vi "New Items.vi"(8 "error in (no error)":errorcluster, 10 "New Items":refnum<class "BetterItem.lvclass">[](array[class]), 11 "BetterTreeHandle in":refnum<class "BetterTreeHandle.lvclass">) -> (0 "error out":errorcluster, 3 "BetterTreeHandle out":refnum<class "BetterTreeHandle.lvclass">)   [LabVIEW 2020, in "BetterDragAndDrop.lvlib" / "BetterTreeHandle.lvclass"]
uses:
  BetterTreeHandle.lvclass
  C:/DSCE code/Open-source/betterdraganddrop_GIT/Source/Classes/BetterHandle/BetterHandle.lvclass
  BetterTreeItem/BetterItem.lvclass
  BetterTreeHandle.lvclass/BetterTreeHandle.ctl
  BetterHandle/BetterHandle.lvclass/BetterHandle.ctl
  BetterHandle/BetterHandle.lvclass
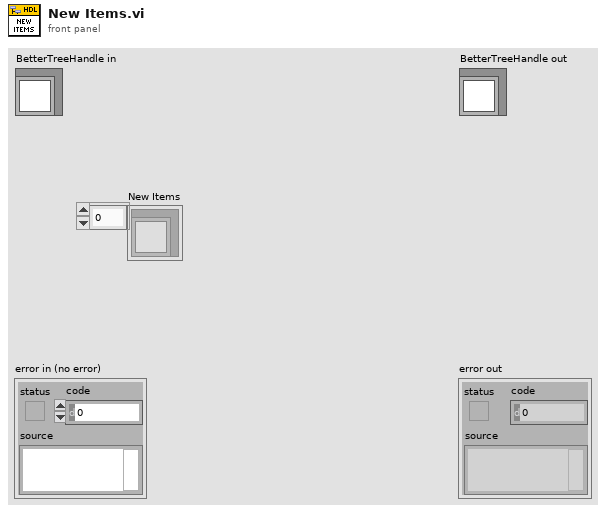
[diagram p1: front panel]
types:
  T1 = cluster{"Left Cell String":string, "Child Text":string[], "Child Tag":string, "Item Indent":i32, "Child Only?":bool, "Glyph Index":i32}
  T2 = typedef "BetterDragAndDrop.lvlib/BetterTreeHandle.lvclass/TreeItem.ctl" = cluster{"Left Cell String":string, "Child Text":string[], "Child Tag":string, "Item Indent":i32, "Child Only?":bool, "Glyph Index":i32, "Font Color":u32}
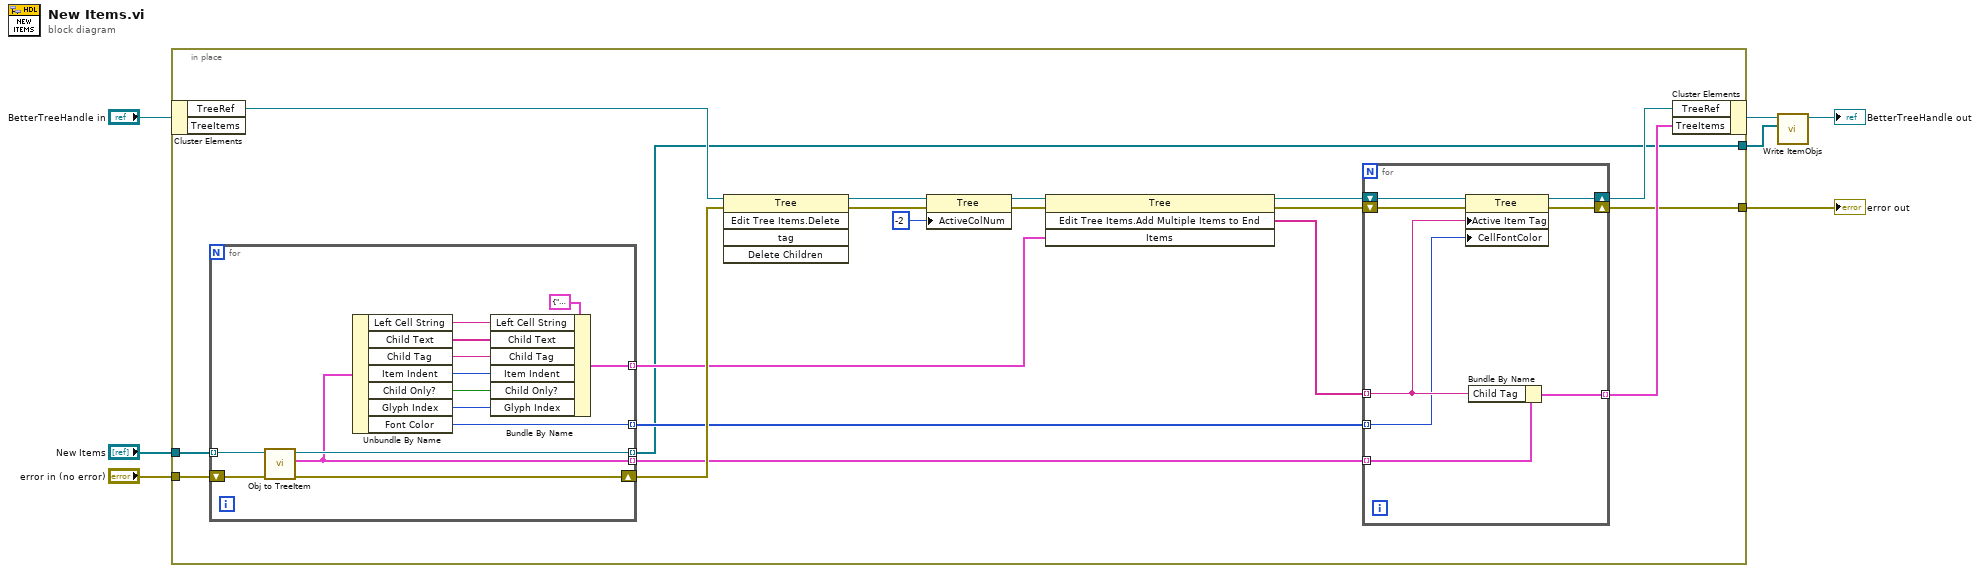
[diagram p0: block diagram]
diagram:
  n1 = in-place {
    in-place-border: "error in (no error)" -> [w25]
    in-place-border: [w10] -> w3
    in-place-border: "New Items" -> [w9]
    in-place-border: [w8] -> w5
    n2 = in-place-cluster #1("BetterTreeHandle in") -> ("TreeRef"=w26:refnum<vi>)  [unwired: 1 out]
    n3 = for {
      tunnel: w9 -> [w31] mode=indexing
      tunnel: [w29] -> w8 mode=indexing
      tunnel: [w27] -> w23 mode=indexing
      shift-right: [w28] -> w24
      shift-left: w25 -> [w30]
      tunnel: [w33] -> w21 mode=indexing
      tunnel: [w32] -> w13 mode=indexing
      n4 = call "Obj to TreeItem.vi"("error in (no error)"=w30, "BetterTreeItem in"=w31) -> ("error out"=w28:errorcluster, "Tree Control Item"=w27:T2, "BetterTreeItem out"=w29:refnum<class "BetterItem.lvclass">)  [unwired: 7 in]
      n5 = Unbundle By Name(w27) -> ("Left Cell String"=w39:string, "Child Text"=w34:string[], "Child Tag"=w35:string, "Item Indent"=w36:i32, "Child Only?"=w37:bool, "Glyph Index"=w38:i32, "Font Color"=w32:u32)
      n6 = Bundle By Name(cluster=T1 {"Left Cell String"="", "Child Text"=[], "Child Tag"="", "Item Indent"=0, "Child Only?"=FALSE, "Glyph Index"=0} ("Item"), "Left Cell String"=w39, "Child Text"=w34, "Child Tag"=w35, "Item Indent"=w36, "Child Only?"=w37, "Glyph Index"=w38) -> (w33:T1)
    }
    n7 = invoke class="Tree" method="Edit Tree Items.Delete"(reference=w26, error in=w24) -> (reference out=w20:refnum<vi>, error out=w18:errorcluster)  [unwired: 3 in, 3 out]
    n8 = property class="Tree"(reference=w20, error in=w18, "ActiveColNum"=-2 ("Active Cell:Active Column Number")) -> (reference out=w17:refnum<vi>, error out=w16:errorcluster)
    n9 = invoke class="Tree" method="Edit Tree Items.Add Multiple Items to End"(reference=w17, error in=w16, "Items"=w21) -> (reference out=w14:refnum<vi>, error out=w12:errorcluster, "Edit Tree Items:Add Multiple Items to End"=w15:string[])  [unwired: 1 in, 1 out]
    n10 = for {
      tunnel: w23 -> [w48] mode=indexing
      tunnel: w15 -> [w45] mode=indexing
      tunnel: [w47] -> w22 mode=indexing
      shift-right: [w43] -> w11
      shift-left: w14 -> [w46]
      tunnel: w13 -> [w44] mode=indexing
      shift-right: [w41] -> w10
      shift-left: w12 -> [w42]
      n11 = property class="Tree"(reference=w46, error in=w42, "Active Item Tag"=w45, "CellFontColor"=w44) -> (reference out=w43:refnum<vi>, error out=w41:errorcluster)
      n12 = Bundle By Name(cluster=w48, "Child Tag"=w45) -> (w47:T2)
    }
    n13 = in-place-cluster #1("TreeRef"=w11, "TreeItems"=w22) -> (w6:refnum<class "BetterTreeHandle.lvclass">)
  }
  "error out" <- w3
  n14 = call "Write ItemObjs.vi"("ItemObjs"=w5, "BetterHandle in"=w6) -> ("BetterHandle out"=→"BetterTreeHandle out":refnum<class "BetterTreeHandle.lvclass">)  [unwired: 9 in]
